vi "To bytes.vi"(3 "MsgPackNil in":refnum<class "MsgPackNil.lvclass">) -> (1 "Array":u8[](array[numeric]))   [LabVIEW 2020, in "MessagePack.lvlib" / "MsgPackNil.lvclass"]
uses:
  MsgPackNil.lvclass
  MsgPackNil.lvclass/MsgPackNil.ctl
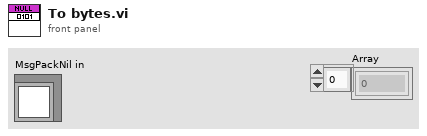
[diagram p1: front panel]
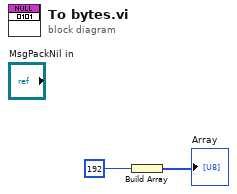
[diagram p0: block diagram]
diagram:
  n1 = Build Array(u8 192) -> (→"Array":u8[])
